vi "Constructor__icon_lib_labview_project_api.vi"(8 "error in (no error)":errorcluster, 10 "Open Window (F)":bool, 11 "Project Path":path) -> (0 "error out":errorcluster, 3 "Project Reference":refnum<vi>)   [LabVIEW 2016, in "LabVIEW Project API__icon_lib_labview_project_api.lvlib"]
doc: "Opens a reference to a Project.\n\n<b>Author:</b> JG\n\n<b>ICON Technologies Pty Ltd</b>\nCopyright (C) 1990-2009\nAll Rights Reserved"
uses:
  LabVIEW Project API__icon_lib_labview_project_api.lvlib
panel:
  # "Output"
  # "Input"
  # "ICON Technologies Pty Ltd\nCopyright (C) 1990-2009\nAll Rights Reserved"
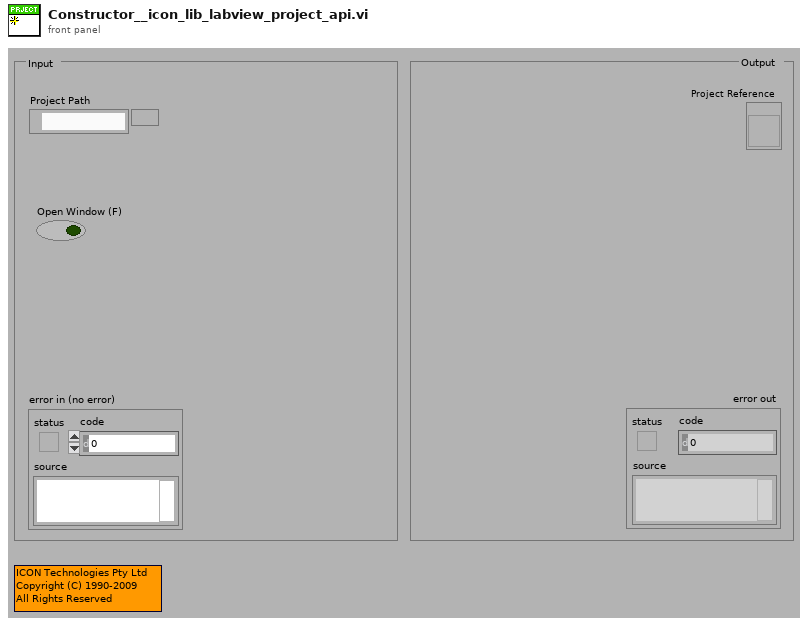
[diagram p1: front panel]
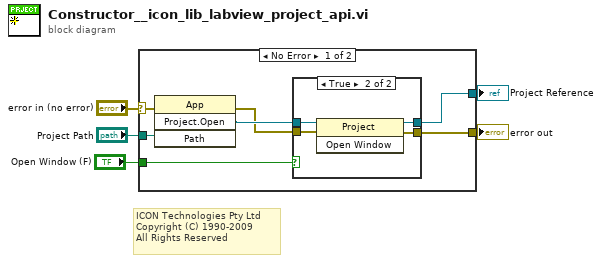
[diagram p0: block diagram]
diagram:
  # "ICON Technologies Pty Ltd\nCopyright (C) 1990-2009\nAll Rights Reserved"
  n1 = case shown="No Error" "error in (no error)" {
    selector: "error in (no error)" -> [w12 w19]
    tunnel: [w7 w19] -> w4
    tunnel: "Project Path" -> [w11 _]
    tunnel: [w9 _] -> w2
    tunnel: "Open Window (F)" -> [w6 _]
    frame No Error {
      n2 = invoke class="App" method="Project.Open"(error in=w12, "Path"=w11) -> (error out=w8:errorcluster, "Project:Open"=w10:refnum<vi>)  [unwired: 2 in, 2 out]
      n3 = case shown="True" w6 {
        tunnel: w10 -> [w14 w18]
        tunnel: [w14 w17] -> w9
        tunnel: w8 -> [w13 w16]
        tunnel: [w13 w15] -> w7
        frame False {
        }
        frame True {
          n4 = invoke class="Project" method="Open Window"(reference=w18, error in=w16) -> (reference out=w17:refnum<vi>, error out=w15:errorcluster)  [unwired: 1 in, 1 out]
        }
      }
    }
    frame Error {
    }
  }
  "error out" <- w4
  "Project Reference" <- w2
